vi "Append Category.vi"(8 "error in (no error)":errorcluster, 10 "name":string, 11 "Database in":refnum<class "Account History.lvclass">) -> (0 "error out":errorcluster, 3 "Database out":refnum<class "Account History.lvclass">)   [LabVIEW 2018, in "Account History.lvclass"]
uses:
  Account History.lvclass
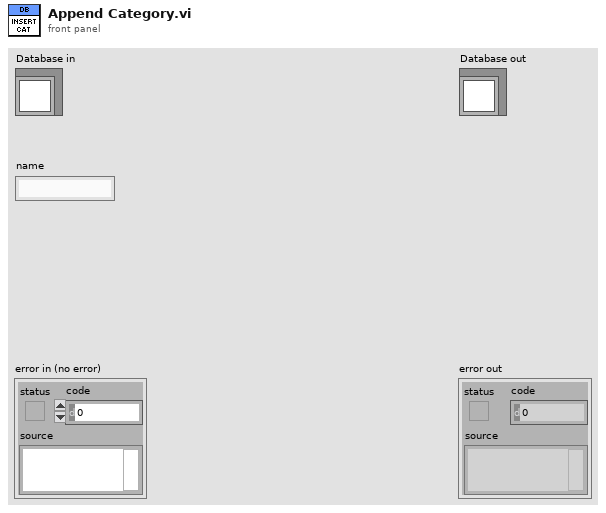
[diagram p1: front panel]
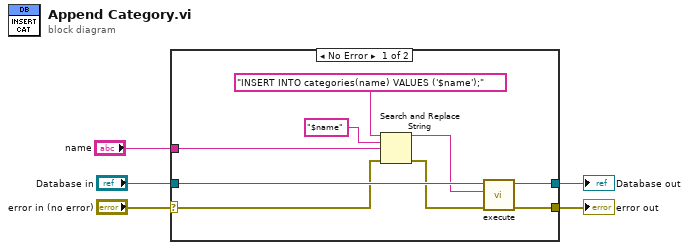
[diagram p0: block diagram]
diagram:
  n1 = case shown="No Error" "error in (no error)" {
    selector: "error in (no error)" -> [w11 w16]
    tunnel: [w12 w16] -> w4
    tunnel: [w13 w15] -> w2
    tunnel: "Database in" -> [w14 w15]
    tunnel: "name" -> [w8 _]
    frame No Error {
      n2 = Search and Replace String(input string="INSERT INTO categories(name) VALUES ('$name');", search string="$name", replace string=w8, error in=w11) -> (result string=w6:string, error out=w10:errorcluster)  [unwired: 4 in, 2 out]
      n3 = call "execute.vi"("error in (no error)"=w10, "SQL query"=w6, "Database in"=w14) -> ("error out"=w12:errorcluster, "Database out"=w13:refnum<class "Account History.lvclass">)  [unwired: 7 in]
    }
    frame Error {
    }
  }
  "error out" <- w4
  "Database out" <- w2
